vi "arreglobidi4.vi"() -> ()   [LabVIEW 2011]
panel:
  out "Array":dbl[][](array[numeric])
  # "ingresar numeros enteros entre 1-200 , luego en la ultima linea del arreglo\nreservarla para obtener el numero mayor de cada una de las columnas."
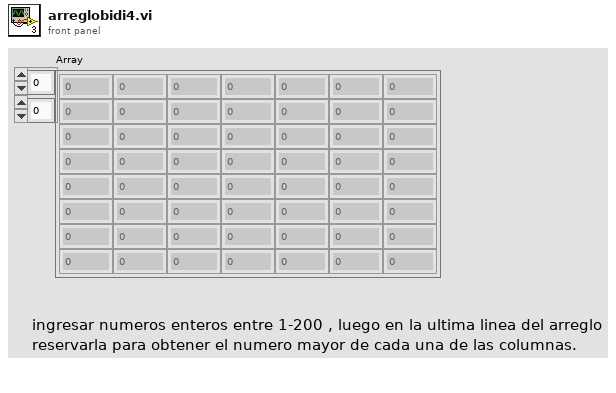
[diagram p1: front panel]
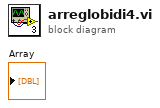
[diagram p0: block diagram]
diagram:
